vi "Main_Fun_Dequeue.vi"(8 "Error in":errorcluster, 11 "Message Queue":refnum<queue>) -> (0 "Error Out":errorcluster, 1 "Queue Data":variant, 2 "Queue Action":T1=enum."動作-系統初始化", 3 "Message Queue Out":refnum<queue>)   [LabVIEW 2015]
uses:
  Control_Main_QData.ctl
  Control_Main_Queue Action.ctl
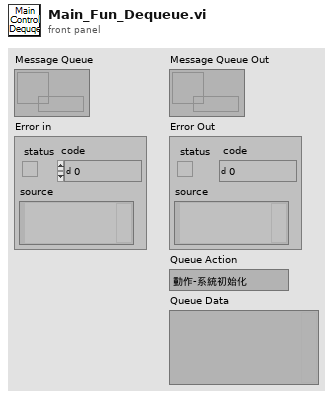
[diagram p1: front panel]
types:
  T1 = typedef "Control_Main_Queue Action.ctl" = enum16{"動作-使用者登入", "動作-系統初始化", "動作-開始", "動作-系統管理選單", "動作-資料管理", "動作-登出/離開", "動作-關於本系統", "1.0 帳號管理", "    1.1 登入", "    1.2 確認狀態", "    1.3 更新介面", "    1.4 帳號管理", "    1.5 登出", "2.0 每日點檢", "10.0 系統", "    10.1 系統-關機", "    10.2 系統-等待", "    10.3 系統-回到作業系統"}
  T2 = typedef "Control_Main_QData.ctl" = cluster{"Queue Action":T1, "Queue Data":variant}
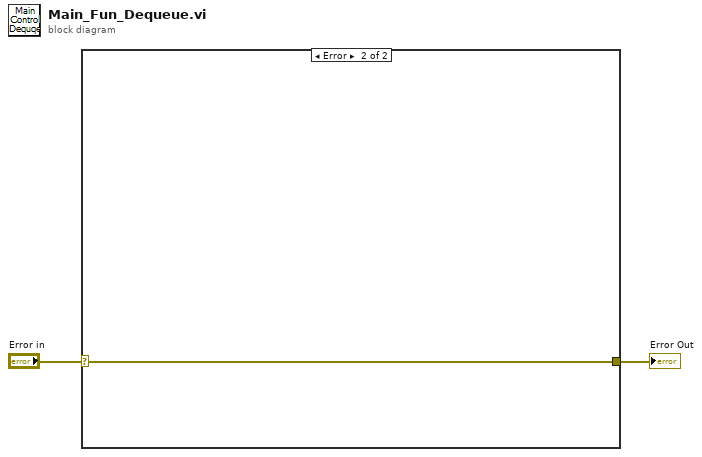
[diagram p0: block diagram]
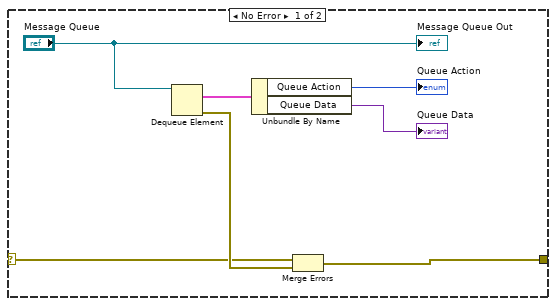
[diagram p2: hidden frame]
diagram:
  n1 = case shown="Error" "Error in" {
    selector: "Error in" -> [w3 w10]
    tunnel: [w4 w10] -> w2
    frame No Error {
      n2 = Dequeue Element(queue="Message Queue") -> (element=w8:T2, error out=w9:errorcluster)  [unwired: 2 in, 2 out]
      n3 = Unbundle By Name(w8) -> ("Queue Action"=→"Queue Action":T1, "Queue Data"=→"Queue Data":variant)
      n4 = Merge Errors(w3, w9) -> (w4:errorcluster)
      "Message Queue Out" <- "Message Queue"
    }
    frame Error {
    }
  }
  "Error Out" <- w2
